vi "UMB_WallAvoid.vi"(9 "behavior weights":i8[](array[numeric]), 10 "Boat Heading":i32, 11 "MapDAR Data (r:pixel b:degrees)":cluster{"Range":dbl, "Bearing":dbl}[](array[cluster])) -> (3 "Behavior Output":T2)   [LabVIEW 2012]
uses:
  NINJA Code/Tugboat/Robo_Programs/behaviorOutput_t.ctl
panel:
  in  "tweakers cluster":T1
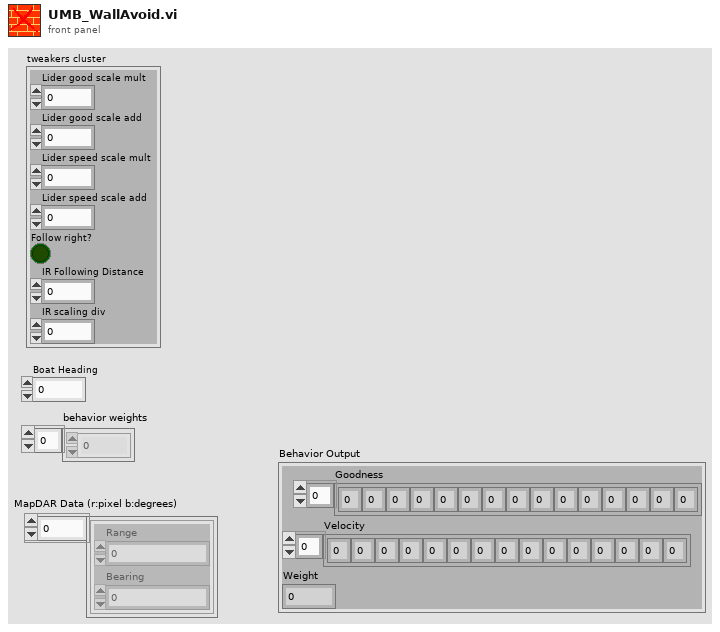
[diagram p1: front panel]
types:
  T1 = cluster{"Lider good scale mult":i32, "Lider good scale add":i32, "Lider speed scale mult":i32, "Lider speed scale add":i32, "Follow right?":bool, "IR Following Distance":i32, "IR scaling div":i32}
  T2 = typedef "behaviorOutput_t.ctl" = cluster{"Goodness":i8[], "Velocity":i8[], "Weight":i8}
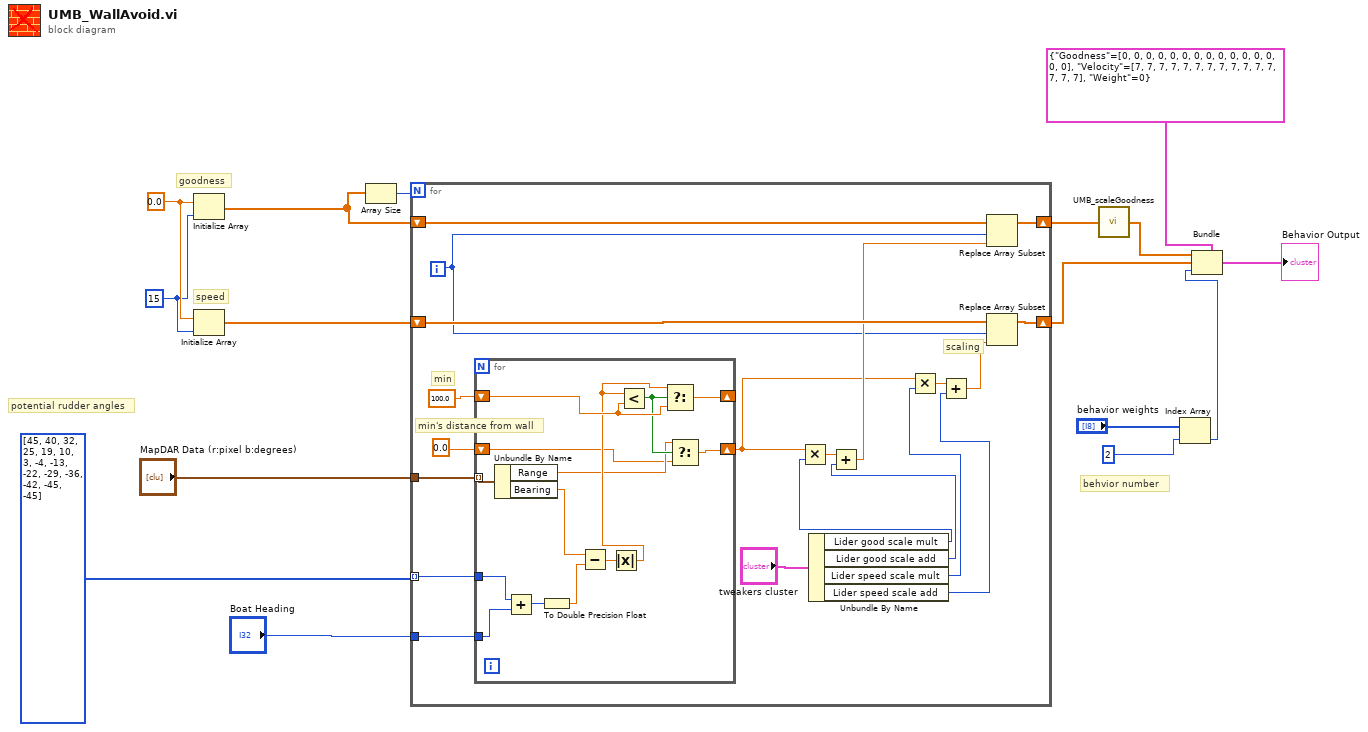
[diagram p0: block diagram]
diagram:
  w15 = 15 ("dimension size")
  w16 = 0.0 ("element")
  # "potential rudder angles"
  # "behvior number"
  # "goodness"
  # "speed"
  n1 = Initialize Array(w16, w15) -> (w14:dbl[])
  n2 = Initialize Array(w16, w15) -> (w13:dbl[])
  n3 = Array Size(array=w14) -> (size(s)=w12:i32)
  n4 = for {
    N: w12 -> [_]
    shift-right: [w34] -> w11
    shift-left: w14 -> [w36]
    shift-right: [w33] -> w7
    shift-left: w13 -> [w35]
    tunnel: i32[] [45, 40, 32, 25, 19, 10, 3, -4, -13, -22, -29, -36, -42, -45, -45] -> [w31] mode=indexing
    tunnel: "Boat Heading" -> [w32]
    tunnel: "MapDAR Data (r:pixel b:degrees)" -> [w30]
    i -> [w22]
    # "scaling"
    # "min's distance from wall"
    # "min"
    n5 = for {
      tunnel: w32 -> [w50]
      tunnel: w31 -> [w49]
      tunnel: w30 -> [w48] mode=indexing
      shift-right: [w43] -> _
      shift-left: 100.0 -> [w42]
      shift-right: [w40] -> w24
      shift-left: 0.0 -> [w37]
      n6 = Unbundle By Name(w48) -> ("Range"=w38:dbl, "Bearing"=w45:dbl)
      n7 = Add(x=w49, y=w50) -> (x+y=w47:i32)
      n8 = To Double Precision Float(number=w47) -> (double precision float=w46:dbl)
      n9 = Subtract(x=w45, y=w46) -> (x-y=w44:dbl)
      n10 = Absolute Value(x=w44) -> (abs(x)=w41:dbl)
      n11 = Less?(x=w41, y=w42) -> (x < y?=w39:bool)
      n12 = Select(t=w41, s=w39, f=w42) -> (s? t:f=w43:dbl)
      n13 = Select(t=w38, s=w39, f=w37) -> (s? t:f=w40:dbl)
    }
    n14 = Unbundle By Name("tweakers cluster") -> ("Lider good scale mult"=w20:i32, "Lider good scale add"=w19:i32, "Lider speed scale mult"=w18:i32, "Lider speed scale add"=w17:i32)
    n15 = Multiply(x=w24, y=w20) -> (x*y=w27:dbl)
    n16 = Add(x=w27, y=w19) -> (x+y=w26:dbl)
    n17 = Multiply(x=w24, y=w18) -> (x*y=w25:dbl)
    n18 = Add(x=w25, y=w17) -> (x+y=w23:dbl)
    n19 = Replace Array Subset(array=w36, new element=w26, index=w22) -> (w34:dbl[])
    n20 = Replace Array Subset(array=w35, new element=w23, index=w22) -> (w33:dbl[])
  }
  n21 = call "UMB_scaleGoodness.vi"("goodness"=w11) -> ("scaled goodness"=w8:dbl[])
  n22 = Index Array(array="behavior weights", index=2) -> (element=w4:i8)
  n23 = Bundle(cluster=T2 {"Goodness"=[0, 0, 0, 0, 0, 0, 0, 0, 0, 0, 0, 0, 0, 0, 0], "Velocity"=[7, 7, 7, 7, 7, 7, 7, 7, 7, 7, 7, 7, 7, 7, 7], "Weight"=0} ("Behavior Output"), "Goodness"=w8, "Velocity"=w7, "Weight"=w4) -> (→"Behavior Output":T2)
